vi "Write Acceleration.vi"(8 "error in (no error)":errorcluster, 10 "Acceleration in":refnum<class "Vector2.lvclass">, 11 "PhysicsComponent in":refnum<class "PhysicsComponent.lvclass">) -> (0 "error out":errorcluster, 3 "PhysicsComponent out":refnum<class "PhysicsComponent.lvclass">)   [LabVIEW 2022 SP3, in "PhysicsComponent.lvclass"]
uses:
  PhysicsComponent.lvclass
  PhysicsComponent.lvclass/PhysicsComponent.ctl
  Math/Vector2/Vector2.lvclass
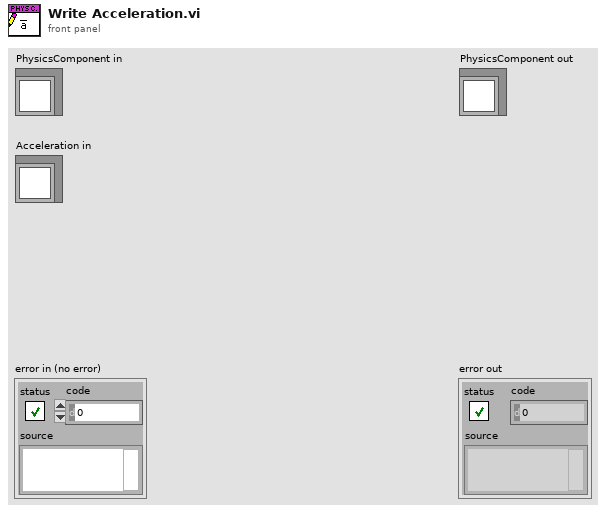
[diagram p1: front panel]
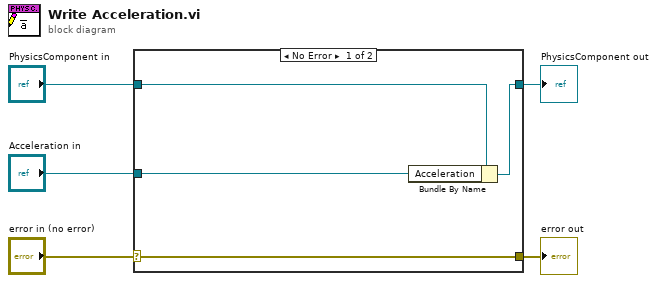
[diagram p0: block diagram]
diagram:
  n1 = case shown="No Error" "error in (no error)" {
    selector: "error in (no error)" -> [w9 w10]
    tunnel: [w9 w10] -> w4
    tunnel: [w7 w11] -> w2
    tunnel: "PhysicsComponent in" -> [w8 w11]
    tunnel: "Acceleration in" -> [w6 _]
    frame No Error {
      n2 = Bundle By Name(cluster=w8, "Acceleration"=w6) -> (w7:refnum<class "PhysicsComponent.lvclass">)
    }
    frame Error {
    }
  }
  "error out" <- w4
  "PhysicsComponent out" <- w2
